vi "Enqueue Action.vi"(8 "error in (no error)":errorcluster, 9 "Data":variant, 10 "Name":T1, 11 "Priority":T2=enum."Interrupt") -> (0 "error out":errorcluster)   [LabVIEW 2014]
uses:
  Action/Action Priority.ctl
  Action/Action Name.ctl
  Action/Action.ctl
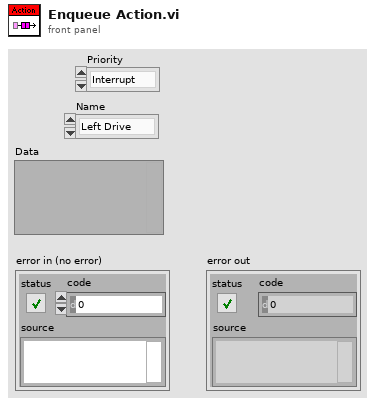
[diagram p1: front panel]
types:
  T1 = typedef "Action Name.ctl" = enum16{"Left Drive", "Right Drive"}
  T2 = typedef "Action Priority.ctl" = enum16{"Normal", "High", "Interrupt"}
  T3 = typedef "Action.ctl" = cluster{"Priority":T2, "Name":T1, "Data":variant}
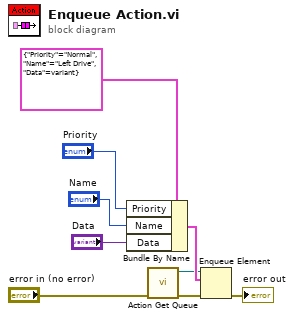
[diagram p0: block diagram]
diagram:
  n1 = Bundle By Name(cluster=T3 {"Priority"=enum."Normal", "Name"=enum."Left Drive", "Data"=variant} ("Action"), "Priority"="Priority", "Name"="Name", "Data"="Data") -> (w6:T3)
  n2 = call "Action Get Queue.vi"("error in (no error)"="error in (no error)") -> ("error out"=w1:errorcluster, "queue out"=w3:refnum<queue>)  [unwired: 9 in]
  n3 = Enqueue Element(queue=w3, element=w6, error in (no error)=w1) -> (error out=→"error out":errorcluster)  [unwired: 1 in, 2 out]
